vi "Read_Graph.vi"() -> (1 "传感器复检":cluster{dbl[], dbl[]}[](graph), 2 "动优化态":cluster{dbl[], dbl[]}[](graph), 3 "动优化态前":cluster{dbl[], dbl[]}[](graph))   [LabVIEW 2020]
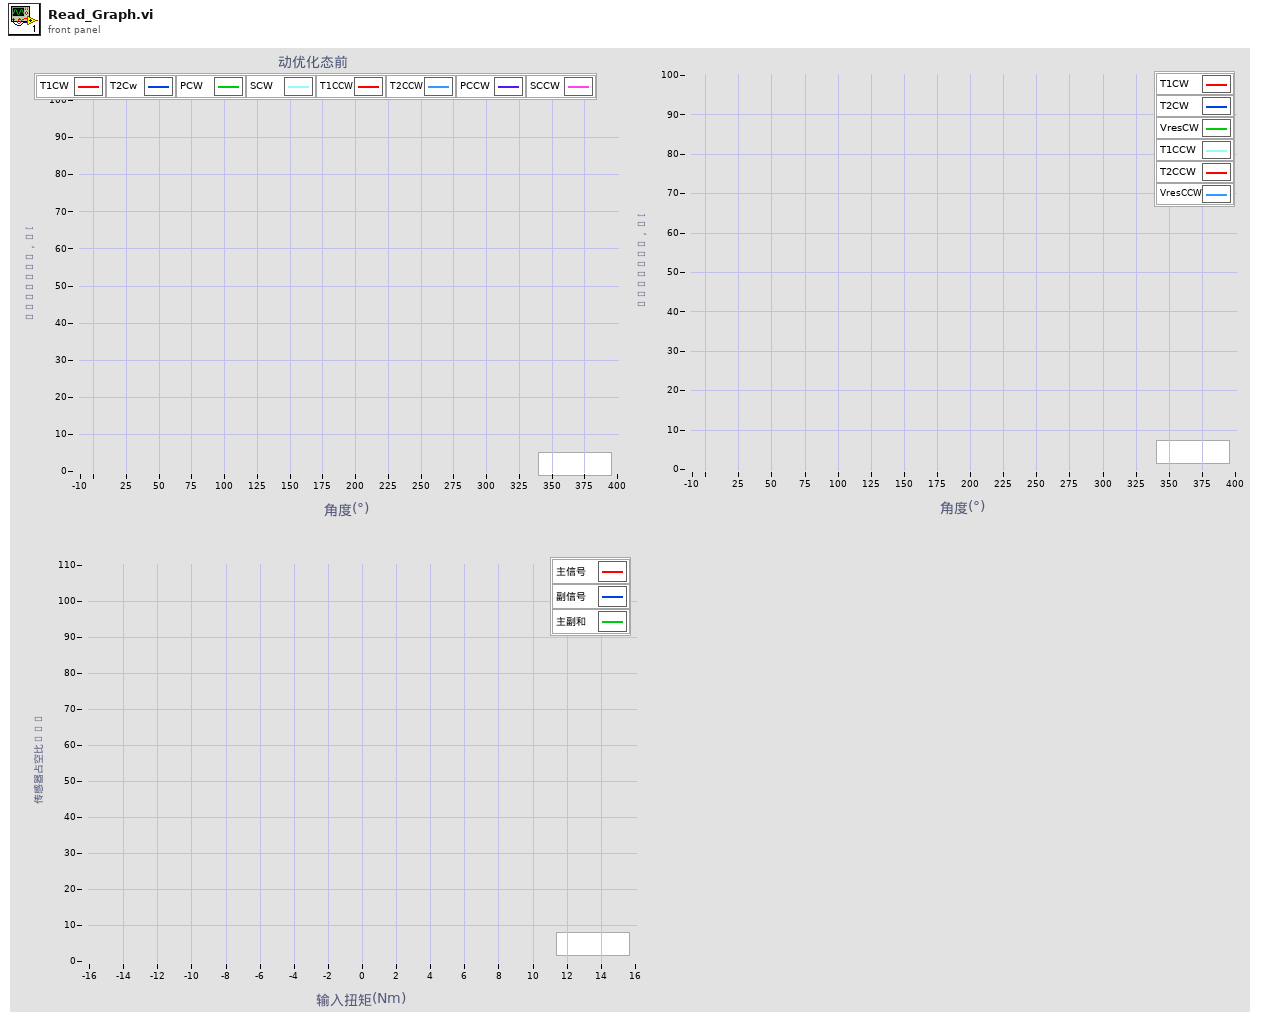
[diagram p1: front panel]
types:
  T1 = enum16{"open", "replace", "create", "open or create", "replace or create", "replace or create with confirmation"}
  T2 = cluster{"动优化态":cluster{dbl[], dbl[]}[], "动优化态前":cluster{dbl[], dbl[]}[], "传感器复检":cluster{dbl[], dbl[]}[]}
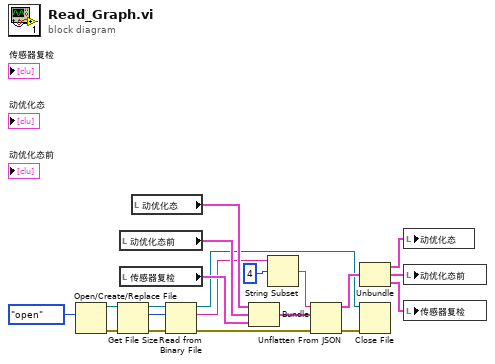
[diagram p0: block diagram]
diagram:
  n1 = Open/Create/Replace File(operation (0:open)=T1."open" ("操作(0:open)")) -> (refnum out=w14:refnum<file>, error out=w13:errorcluster)  [unwired: 5 in, 1 out]
  n2 = Get File Size(file=w14, error in=w13) -> (refnum out=w2:refnum<file>, size (in bytes)=w15:i64, 0:w16:errorcluster)
  n3 = local read "动优化态前"() -> (w19:cluster{dbl[], dbl[]}[])
  n4 = local read "传感器复检"() -> (w17:cluster{dbl[], dbl[]}[])
  n5 = local read "动优化态"() -> (w20:cluster{dbl[], dbl[]}[])
  n6 = Read from Binary File(8:w16, 10:w15, 11:w2) -> (0:w11:errorcluster, 2:w12:string, 3:w3:refnum<file>)  [unwired: 3 in, 1 out]
  n7 = Bundle("动优化态"=w20, "动优化态前"=w19, "传感器复检"=w17) -> (w9:T2)  [unwired: 1 in]
  n8 = String Subset(string=w12, offset (0)=4 ("长度（剩余）")) -> (substring=w10:string)  [unwired: 1 in]
  n9 = Unflatten From JSON(JSON string=w10, type and defaults=w9, error in (no error)=w11) -> (value=w8:T2, error out=w4:errorcluster)  [unwired: 4 in]
  n10 = Unbundle(w8) -> ("动优化态"=w7:cluster{dbl[], dbl[]}[], "动优化态前"=w6:cluster{dbl[], dbl[]}[], "传感器复检"=w5:cluster{dbl[], dbl[]}[])
  n11 = Close File(refnum=w3, error in=w4) -> ()  [unwired: 2 out]
  n12 = local write "动优化态"(w7) -> ()
  n13 = local write "动优化态前"(w6) -> ()
  n14 = local write "传感器复检"(w5) -> ()
